vi "Reset PMTs.vi"(8 "Error In":errorcluster) -> (0 "Error Out":errorcluster)   [LabVIEW 2020]
uses:
  <vilib>/DAQmx/write.llb/DAQmx Write (Analog 1D DBL NChan 1Samp).vi
  <vilib>/DAQmx/create/channels.llb/DAQmx Create Channel (AO-Voltage-Basic).vi
  <vilib>/DAQmx/miscellaneous.llb/DAQmx Fill In Error Info.vi
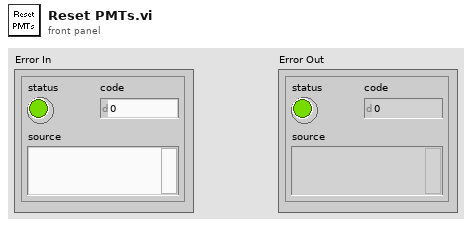
[diagram p1: front panel]
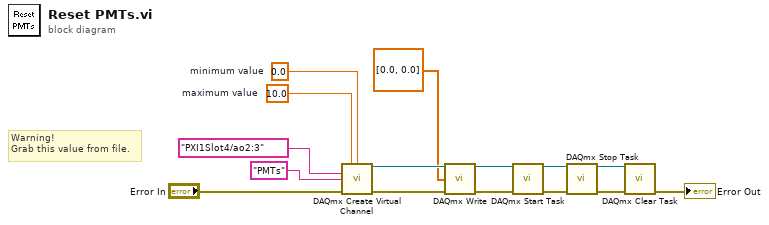
[diagram p0: block diagram]
diagram:
  w6 = 10.0  # maximum value
  w7 = 0.0  # minimum value
  # "Warning!\nGrab this value from file."
  n1 = call-poly <vilib>:"DAQmx Create Virtual Channel.vi"("maximum value"=w6, "minimum value"=w7, "physical channels"=tag "PXI1Slot4/ao2:3" ("DAQmx Physical Channel"), "name to assign"="PMTs", "error in"="Error In") -> ("task out"=w15:refnum<k21>, "error out"=w14:errorcluster)  [unwired: 9 in]
  n2 = call-poly <vilib>:"DAQmx Write.vi"("task/channels in"=w15, "data"=dbl[] [0.0, 0.0], "error in"=w14) -> ("task out"=w13:refnum<k21>, "error out"=w12:errorcluster)  [unwired: 10 in, 1 out]
  n3 = call <vilib>:"DAQmx Start Task.vi"("task/channels in"=w13, "error in"=w12) -> ("task out"=w4:refnum<k21>, "error out"=w5:errorcluster)  [unwired: 12 in]
  n4 = call <vilib>:"DAQmx Stop Task.vi"("task/channels in"=w4, "error in"=w5) -> ("task out"=w11:refnum<k21>, "error out"=w10:errorcluster)  [unwired: 12 in]
  n5 = call <vilib>:"DAQmx Clear Task.vi"("task in"=w11, "error in"=w10) -> ("error out"=→"Error Out":errorcluster)  [unwired: 13 in]
